vi "find_newest_file.vi"(10 "Directory Path to Start the Search":path) -> (0 "Number of Files":i32, 2 "Most Recent File Path":path)   [LabVIEW 2010]
doc: "This program finds all the files in a specified directory and then compares the last modified date and time for each file to find the most recently modified file. The for loop passes the index of the most current file and the array of file paths is indexed to get the file path of the most current file in the directory."
panel:
  out "List of All the File Names":string[](array[string])
  # "- Select the directory path to start the search\n- Run the VI\n- The most recent file in the directory is displayed\n- List of All the File Names array contains the first-level files in the directory"
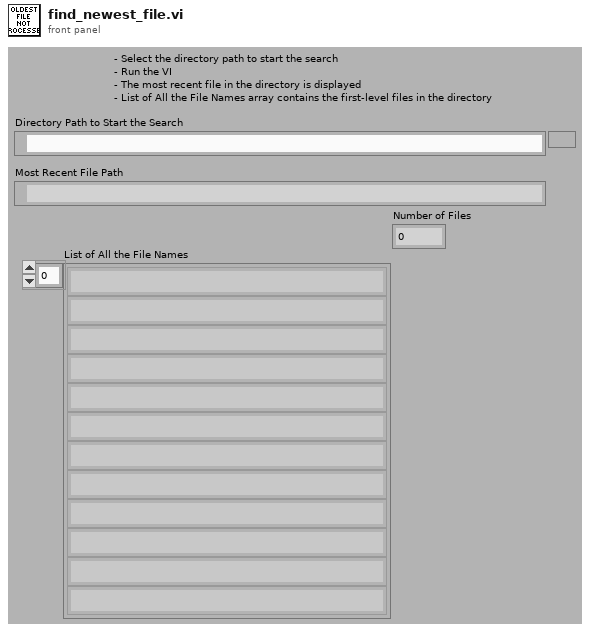
[diagram p1: front panel]
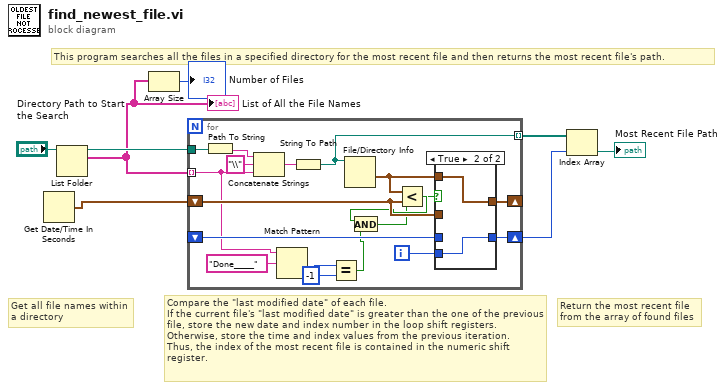
[diagram p0: block diagram]
diagram:
  # "Return the most recent file from the array of found files"
  # "Compare the \"last modified date\" of each file. \nIf the current file's \"last modified date\" is greater than the one of the previous file, store the new date and index number in the loop shift registers. \nOtherwise, store the time and index values from the previous iteration.\nThus, the index of the most recent file is contained in the numeric shift register."
  # "This program searches all the files in a specified directory for the most recent file and then returns the most recent file's path."
  # "Get all file names within a directory"
  n1 = Get Date/Time In Seconds() -> (seconds since 1Jan1904=w3:timestamp)
  n2 = List Folder(path="Directory Path to Start the Search") -> (path out=w8:path, filenames=w2:string[])  [unwired: 3 in, 2 out]
  "List of All the File Names" <- w2
  n3 = Array Size(array=w2) -> (size(s)=→"Number of Files":i32)
  n4 = for {
    tunnel: w8 -> [w26]
    tunnel: w2 -> [w14] mode=indexing
    tunnel: [w22] -> w6 mode=indexing
    shift-right: [w18] -> _
    shift-left: w3 -> [w16]
    shift-right: [w20] -> w4
    shift-left: _ -> [w19]
    i -> [w21]
    n5 = Path To String(path=w26) -> (string=w25:string)
    n6 = Concatenate Strings(w25, "\\" ("string"), w14) -> (w24:string)
    n7 = Match Pattern(string=w14, regular expression="Done_____") -> (offset past match=w12:i32)  [unwired: 1 in, 3 out]
    n8 = String To Path(string=w24) -> (path=w22:path)
    n9 = Equal?(x=w12, y=-1) -> (x = y?=w10:bool)
    n10 = File/Directory Info(path=w22) -> (last mod=w17:timestamp)  [unwired: 1 in, 6 out]
    n11 = Less?(x=w17, y=w16) -> (x < y?=w13:bool)
    n12 = And(x=w13, y=w10) -> (x .and. y?=w9:bool)
    n13 = case shown="True" w9 {
      tunnel: w17 -> [_ w30]
      tunnel: [w27 w30] -> w18
      tunnel: w21 -> [_ w29]
      tunnel: w16 -> [w27 _]
      tunnel: [w28 w29] -> w20
      tunnel: w19 -> [w28 _]
      frame False {
      }
      frame True {
      }
    }
  }
  n14 = Index Array(array=w6, index=w4) -> (element=→"Most Recent File Path":path)
